vi "Test Config.vi"   [LabVIEW 2012]
uses:
  <vilib>/Utility/config.llb/NI_LVConfig.lvlib
types:
  T1 = typedef "NI_LVConfig.lvlib/Config Data RefNum.ctl" = refnum<k1>
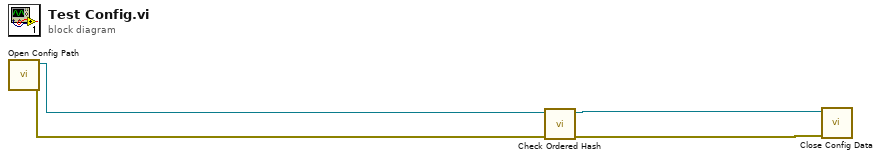
[diagram p0: block diagram]
diagram:
  n1 = call "Open Config Path.vi"() -> ("error out"=w3:errorcluster, "cfg_ref out"=w4:T1)  [unwired: 10 in]
  n2 = call "Check Ordered Hash.vi"("error in"=w3, "refnum"=w4) -> ("error out"=w1:errorcluster, "refnum out"=w2:T1)  [unwired: 6 in, 2 out]
  n3 = call <vilib>:"Close Config Data.vi"("error in (no error)"=w1, "refnum"=w2) -> ()  [unwired: 8 in, 2 out]
